vi "setGlobalLogLevel.vi"(8 "error in (no error)":errorcluster, 10 "LogLevel (daqLogLevelOff)":T1=enum."daqLogLevelOff", 11 "IInstanceBuilder in":refnum<class "IInstanceBuilder.lvclass">) -> (0 "error out":errorcluster, 3 "IInstanceBuilder out":refnum<class "IInstanceBuilder.lvclass">)   [LabVIEW 2022 SP3, in "openDAQ.lvlib" / "IBaseObject.lvlib" / "IInstanceBuilder.lvlib" / "IInstanceBuilder.lvclass"]
uses:
  <instrlib>/openDAQ/Public/Classes/IInstanceBuilder/IInstanceBuilder.lvclass
  C:/Program Files (x86)/National Instruments/LabVIEW 2022/instr.lib/openDAQ/Public/Classes/IBaseObject/IBaseObject.lvclass
  <instrlib>/openDAQ/Public/Classes/ILogger/TypeDef/LogLevel.ctl
  <instrlib>/openDAQ/Public/Classes/IBaseObject/IBaseObject.lvclass/IBaseObject.ctl
  <instrlib>/openDAQ/Public/Classes/IBaseObject/Accessor/Read reference.vi
  <instrlib>/openDAQ/Public/Classes/IBaseObject/Accessor/Write reference.vi
  <instrlib>/openDAQ/Binaries/Windows/x86/copendaq32.dll
  <instrlib>/openDAQ/Public/Classes/ILogger/ILogger.lvclass
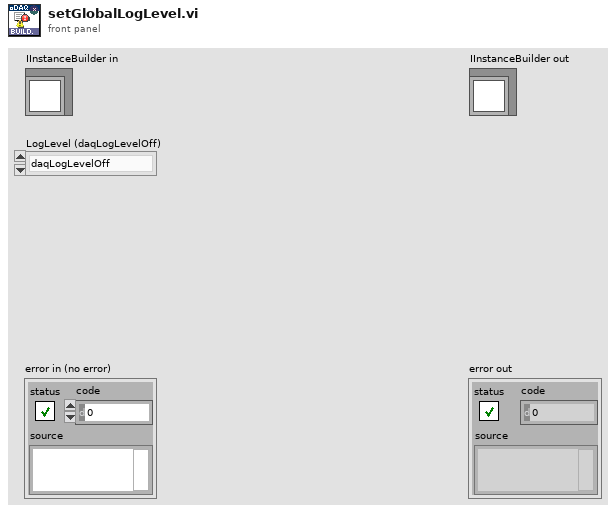
[diagram p1: front panel]
types:
  T1 = typedef "openDAQ.lvlib/IBaseObject.lvlib/ILogger.lvlib/ILogger.lvclass/LogLevel.ctl" = enum16{"daqLogLevelTrace", "daqLogLevelDebug", "daqLogLevelInfo", "daqLogLevelWarn", "daqLogLevelError", "daqLogLevelCritical", "daqLogLevelOff", "daqLogLevelDefault"}
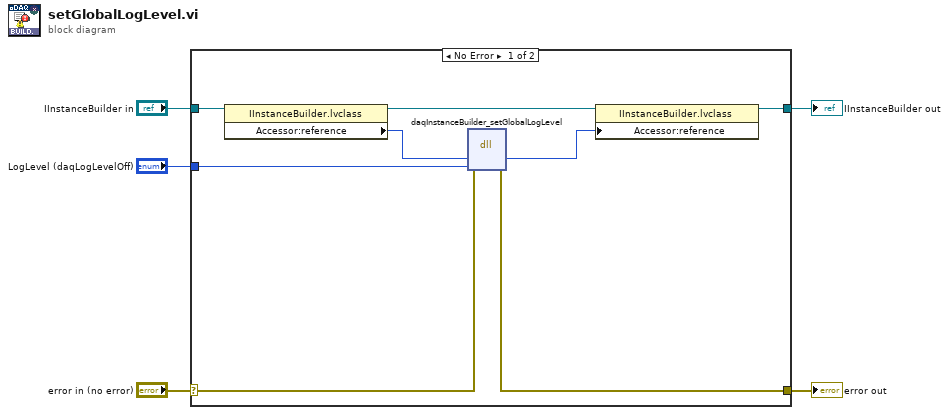
[diagram p0: block diagram]
diagram:
  n1 = case shown="No Error" "error in (no error)" {
    selector: "error in (no error)" -> [w7 w15]
    tunnel: [w6 w15] -> w4
    tunnel: [w11 w14] -> w2
    tunnel: "IInstanceBuilder in" -> [w12 w14]
    tunnel: "LogLevel (daqLogLevelOff)" -> [w13 _]
    frame No Error {
      n2 = property class="IInstanceBuilder.lvclass"(reference=w12) -> (reference out=w10:refnum<class "IInstanceBuilder.lvclass">, "Accessor:reference"=w8:i64)  [unwired: 1 in, 1 out]
      n3 = dll-call lib="C:/Program Files (x86)/National Instruments/LabVIEW 2022/instr.lib/openDAQ/Binaries/Windows/x86/copendaq*.*" fn="daqInstanceBuilder_setGlobalLogLevel"(error in=w7, "instanceBuilder"=w8, "daqLogLevel"=w13) -> (error out=w6:errorcluster, "instanceBuilder"=w9:i64)  [unwired: 4 in, 1 out]
      n4 = property class="IInstanceBuilder.lvclass"(reference=w10, "Accessor:reference"=w9) -> (reference out=w11:refnum<class "IInstanceBuilder.lvclass">)  [unwired: 1 in, 1 out]
    }
    frame Error {
    }
  }
  "error out" <- w4
  "IInstanceBuilder out" <- w2
